vi "Filter Data.vi"(8 "error in (no error)":errorcluster, 10 "Debug Data In":refnum<class "Debug Data.lvclass">[](array[class]), 11 "Filter by Process in":refnum<class "Filter by Process.lvclass">) -> (0 "error out":errorcluster, 2 "Debug Data Out":refnum<class "Debug Data.lvclass">[](array[class]), 3 "Filter by Process out":refnum<class "Filter by Process.lvclass">)   [LabVIEW 2020, in "Filter by Process.lvclass"]
uses:
  Filter by Process.lvclass
  Debug Data/Debug Data.lvclass
  Filter by Process.lvclass/Filter by Process.ctl
  Debug Data/Debug Data.lvclass/Debug Data.ctl
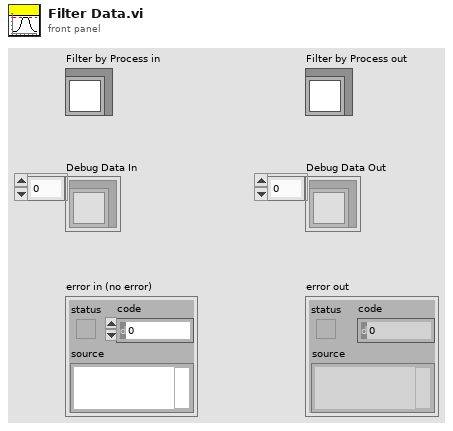
[diagram p1: front panel]
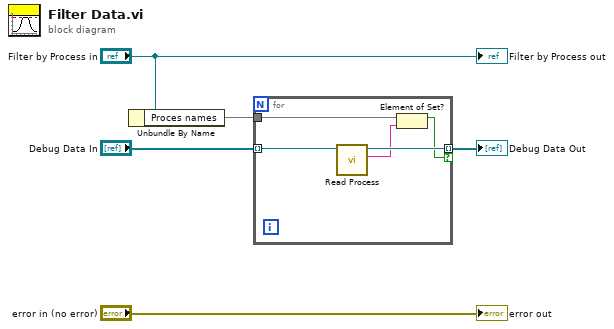
[diagram p0: block diagram]
diagram:
  n1 = Unbundle By Name("Filter by Process in") -> ("Proces names"=w1:set{string})
  n2 = for {
    tunnel: [w9] -> w3 mode=indexing if=w6
    tunnel: "Debug Data In" -> [w10] mode=indexing
    tunnel: w1 -> [w8]
    n3 = call "Read Process.vi"("Debug Data In"=w10) -> ("Process"=w7:string, "Debug Data Out"=w9:refnum<class "Debug Data.lvclass">)  [unwired: 8 in, 1 out]
    n4 = Element of Set?(10:w7, 11:w8) -> (3:w6:bool)
  }
  "Debug Data Out" <- w3
  "error out" <- "error in (no error)"
  "Filter by Process out" <- "Filter by Process in"
